vi "WebDav_main.vi"(8 "error in (no error)":errorcluster caption="Fehler (Eingang, kein Fehler)") -> (0 "error out":errorcluster caption="Fehler (Ausgang)")   [LabVIEW 2020, in "FTP WebDAV.lvlib"]
uses:
  FTP WebDAV.lvlib
  SysLog/SysLog Interface.ctl
  SysLog/SysLog.lvlib
  <vilib>/Utility/Data Type/NI_Data Type.lvlib
  Aktionen FTP WebDAV.ctl
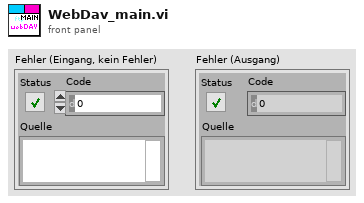
[diagram p1: front panel]
types:
  T1 = typedef "FTP WebDAV.lvlib/Aktionen FTP WebDAV.ctl" = enum16{"lesen", "erkennen"}
  T2 = typedef "FTP WebDAV.lvlib/Enum FTP WebDAV.ctl" = enum16{" nix", "ftp", "webDAV"}
  T3 = typedef "SysLog.lvlib/SysLog Interface.ctl" = cluster{"FehlermeldungsCode":i32, "ErfolgsmeldungsCode":i32, "ParameterListenString":string, "Anzeige":bool, "SysLogIcon":enum16{"OK", "Warnung", "Fehler"}, "intern":bool}
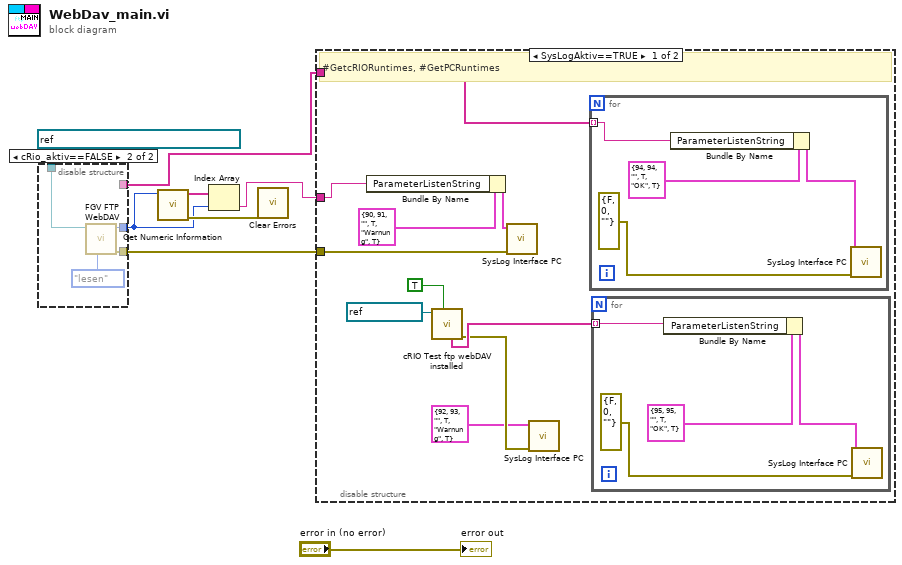
[diagram p0: block diagram]
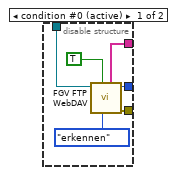
[diagram p2: hidden frame]
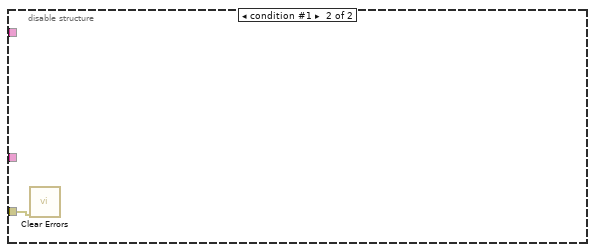
[diagram p3: hidden frame]
diagram:
  n1 = disable-structure shown="cRio_aktiv==FALSE" {
    disable-tunnel: [w13 w17] -> w2
    disable-tunnel: refnum<k21> "NI-cRIO-9066-IAG (192.168.14.14)" ("System Session Ref") -> [w11 w16]
    disable-tunnel: [w10 w15] -> w5
    disable-tunnel: [w9 _] -> w1
    frame condition #0 (active) {
      n2 = call "FGV FTP WebDAV.vi"("Aktionen"=Aktionen_FTP_WebDAV."erkennen", "native Error"=TRUE, "System Session Ref"=w11) -> ("Fehler (Ausgang)"=w13:errorcluster, "ftp webDAV"=w10:T2, "Runtimes"=w9:string[])  [unwired: 4 in, 2 out]
    }
    frame condition #1 {
      n3 = call "FGV FTP WebDAV.vi"("Aktionen"=Aktionen_FTP_WebDAV."lesen", "System Session Ref"=w16) -> ("Fehler (Ausgang)"=w17:errorcluster, "ftp webDAV"=w15:T2)  [unwired: 5 in, 3 out]
    }
  }
  n4 = call <vilib>:"Get Numeric Information.vi"("variant"=w5) -> ("error out"=w6:errorcluster, "enum names"=w4:string[])  [unwired: 7 in, 2 out]
  n5 = Index Array(array=w4, index=w5) -> (element=w7:string)
  n6 = call <vilib>:"Clear Errors.vi"("error in (no error)"=w6) -> ()  [unwired: 5 in, 2 out]
  n7 = disable-structure shown="SysLogAktiv==TRUE" {
    disable-tunnel: w2 -> [w28 w37]
    disable-tunnel: w7 -> [w20 _]
    disable-tunnel: w1 -> [w27 _]
    frame condition #0 (active) {
      # "#GetcRIORuntimes, #GetPCRuntimes"
      n8 = Bundle By Name(cluster=T3 {"FehlermeldungsCode"=90, "ErfolgsmeldungsCode"=91, "ParameterListenString"="", "Anzeige"=TRUE, "SysLogIcon"=enum."Warnung", "intern"=TRUE} ("Cluster (in)"), "ParameterListenString"=w20) -> (w21:T3)
      n9 = call "cRIO Test ftp webDAV installed.vi"("PC"=TRUE, "System Session Ref"=refnum<k21> "localhost") -> ("error out"=w24:errorcluster, "Runtimes"=w25:string[])  [unwired: 6 in, 2 out]
      n10 = call "SysLog Interface PC.vi"("Fehler (in)"=w28, "Cluster (in)"=w21) -> ()  [unwired: 9 in, 1 out]
      n11 = call "SysLog Interface PC.vi"("Fehler (in)"=w24, "Cluster (in)"=T3 {"FehlermeldungsCode"=92, "ErfolgsmeldungsCode"=93, "ParameterListenString"="", "Anzeige"=TRUE, "SysLogIcon"=enum."Warnung", "intern"=TRUE}) -> ()  [unwired: 9 in, 1 out]
      n12 = for {
        tunnel: w27 -> [w33] mode=indexing
        n13 = Bundle By Name(cluster=T3 {"FehlermeldungsCode"=94, "ErfolgsmeldungsCode"=94, "ParameterListenString"="", "Anzeige"=TRUE, "SysLogIcon"=enum."OK", "intern"=TRUE} ("Cluster (in)"), "ParameterListenString"=w33) -> (w34:T3)
        n14 = call "SysLog Interface PC.vi"("Fehler (in)"=errorcluster {"status"=FALSE, "code"=0, "source"=""}, "Cluster (in)"=w34) -> ()  [unwired: 9 in, 1 out]
      }
      n15 = for {
        tunnel: w25 -> [w29] mode=indexing
        n16 = Bundle By Name(cluster=T3 {"FehlermeldungsCode"=95, "ErfolgsmeldungsCode"=95, "ParameterListenString"="", "Anzeige"=TRUE, "SysLogIcon"=enum."OK", "intern"=TRUE} ("Cluster (in)"), "ParameterListenString"=w29) -> (w30:T3)
        n17 = call "SysLog Interface PC.vi"("Fehler (in)"=errorcluster {"status"=FALSE, "code"=0, "source"=""}, "Cluster (in)"=w30) -> ()  [unwired: 9 in, 1 out]
      }
    }
    frame condition #1 {
      n18 = call <vilib>:"Clear Errors.vi"("error in (no error)"=w37) -> ()  [unwired: 5 in, 2 out]
    }
  }
  "error out" <- "error in (no error)"
